vi "set enable value in a cluster.vi"(9 "name":string, 10 "Value":bool, 11 "Clust Refnum":refnum<vi>) -> ()   [LabVIEW 2015]
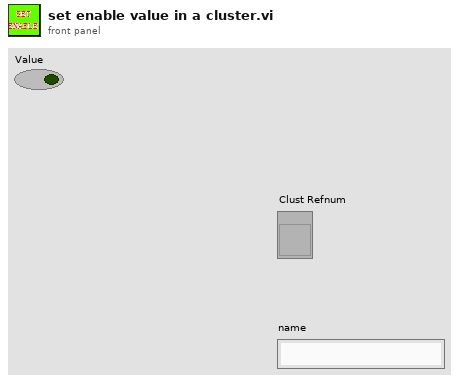
[diagram p1: front panel]
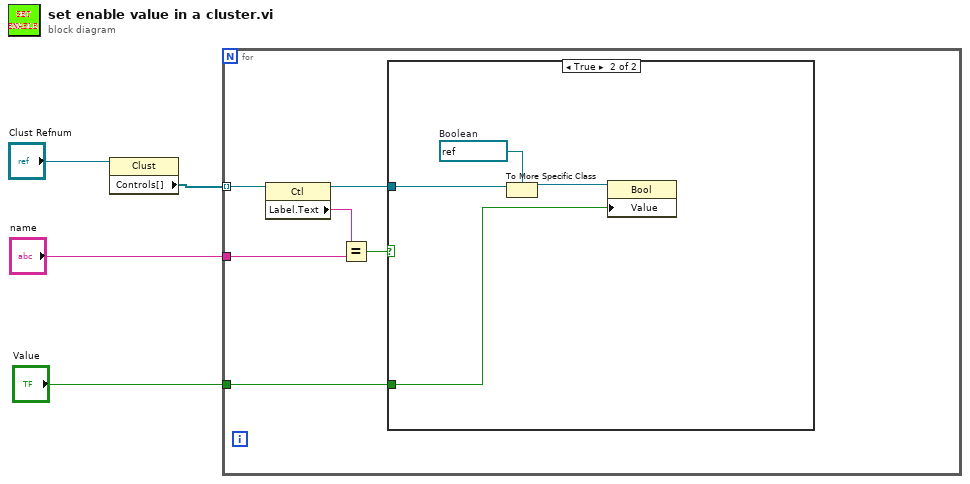
[diagram p0: block diagram]
diagram:
  n1 = property class="Clust"(reference="Clust Refnum") -> ("Controls[]"=w3:refnum<vi>[])  [unwired: 1 in, 2 out]
  n2 = for {
    tunnel: w3 -> [w10] mode=indexing
    tunnel: "name" -> [w8]
    tunnel: "Value" -> [w5]
    n3 = property class="Ctl"(reference=w10) -> (reference out=w6:refnum<vi>, "Label.Text"=w9:string)  [unwired: 1 in, 1 out]
    n4 = Equal?(x=w9, y=w8) -> (x = y?=w7:bool)
    n5 = case shown="True" w7 {
      tunnel: w6 -> [_ w14]
      tunnel: w5 -> [_ w11]
      frame False {
      }
      frame True {
        w13 = refnum<vi> refnum  # Boolean
        n6 = To More Specific Class(target class=w13, reference=w14) -> (specific class reference=w12:refnum<vi>)  [unwired: 1 in, 1 out]
        n7 = property class="Bool"(reference=w12, "Value"=w11) -> ()  [unwired: 1 in, 2 out]
      }
    }
  }
